vi "HVACmotes.vi"() -> ()   [LabVIEW 2011]
uses:
  <vilib>/picture/picture.llb/Draw True-Color Pixmap.vi
panel:
  out "CO2":dbl(graph)
  out "Node ID":u8
  out "Light":dbl(graph)
  out "Humidity":dbl(graph)
  out "Temperature":dbl(graph)
  in  "header size":i32=9
  in  "bytes to read":i32=10
  out "Packet Payload":string
  in  "Enable Read":bool=TRUE
  in  "Port Number":i32=9002
  out "KTH  Automatic Control \nTemplates. Read from SerialForwarder":picture
  # "For TestSerialCommMsg:\nheaderSize = 9\npayload = 10"
  # "Communication control"
  # "Communication results"
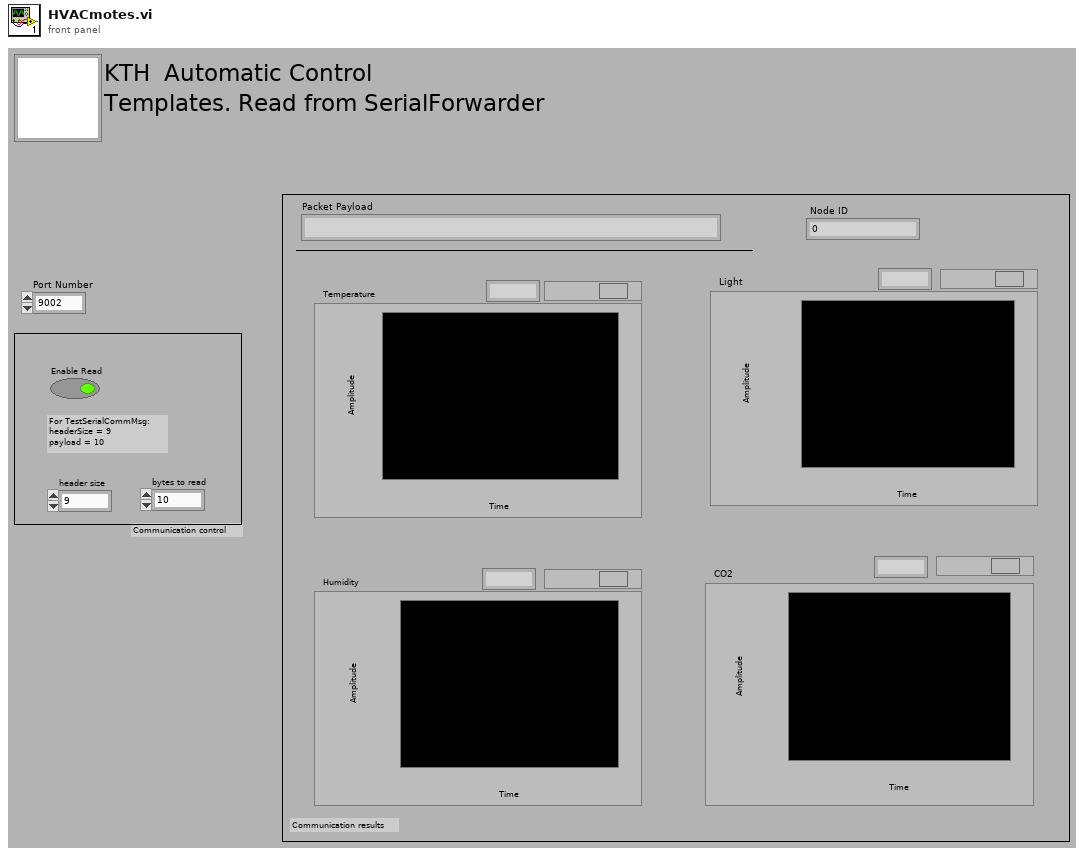
[diagram p1: front panel]
types:
  T1 = typedef "imagedata.ctl" = cluster{"image type":i32, "image depth":i32, "image":u8[], "mask":u8[], "colors":u32[], "Rectangle":cluster{"left":i16, "top":i16, "right":i16, "bottom":i16}}
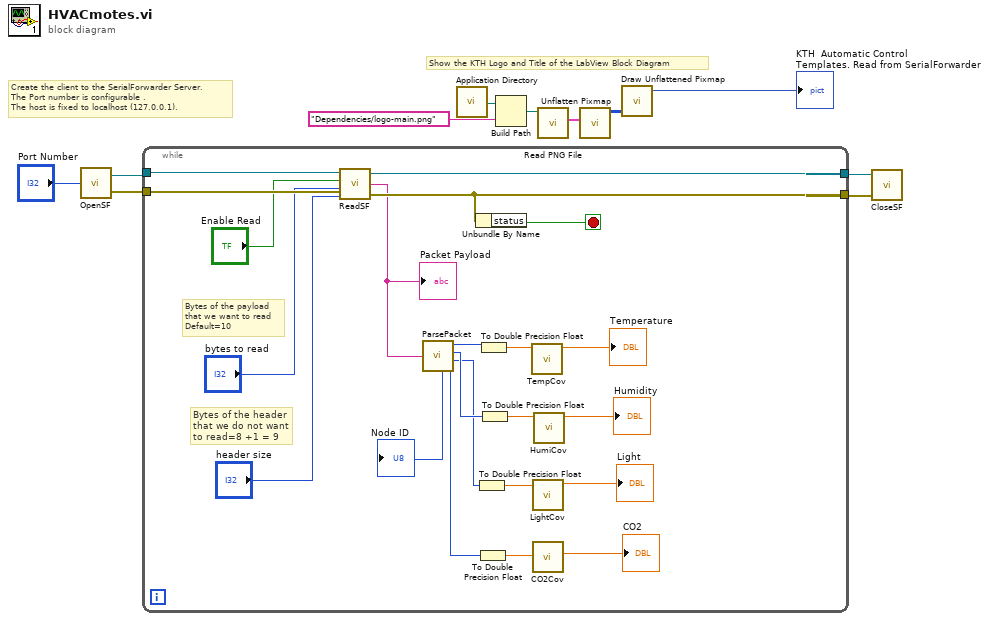
[diagram p0: block diagram]
diagram:
  # "Create the client to the SerialForwarder Server.\nThe Port number is configurable . \nThe host is fixed to localhost (127.0.0.1)."
  # "Show the KTH Logo and Title of the LabView Block Diagram"
  n1 = call "OpenSF.vi"("Port Number"="Port Number") -> ("error out"=w10:errorcluster, "connection ID"=w11:refnum<k5>)
  n2 = while {
    tunnel: w11 -> [w32]
    tunnel: w10 -> [w33]
    tunnel: [w31] -> w9
    tunnel: [w29] -> w8
    stop <- w30 stop-if-true
    # "Bytes of the payload \nthat we want to read\nDefault=10"
    # "Bytes of the header\nthat we do not want \nto read=8 +1 = 9"
    n3 = call "ReadSF.vi"("connection ID in"=w32, "error in"=w33, "enabled"="Enable Read", "bytes to read"="bytes to read", "header size"="header size") -> ("connection ID out"=w31:refnum<k5>, "string"=w25:string, "error out"=w29:errorcluster)  [unwired: 1 in]
    "Packet Payload" <- w25
    n4 = call "ParsePacket.vi"("data out"=w25) -> ("Node ID"=→"Node ID":u8, "CO2"=w15:u16, "Light"=w16:u16, "Humidity"=w17:u16, "Temperature"=w24:u16)  [unwired: 1 out]
    n5 = Unbundle By Name(w29) -> ("status"=w30:bool)
    n6 = To Double Precision Float(number=w16) -> (double precision float=w19:dbl)
    n7 = To Double Precision Float(number=w15) -> (double precision float=w14:dbl)
    n8 = To Double Precision Float(number=w24) -> (double precision float=w23:dbl)
    n9 = To Double Precision Float(number=w17) -> (double precision float=w21:dbl)
    n10 = call "TempCov.vi"("Input x"=w23) -> ("Temperature"=→"Temperature":dbl)  [unwired: 10 in]
    n11 = call "LightCov.vi"("Input x"=w19) -> ("Light"=→"Light":dbl)  [unwired: 10 in]
    n12 = call "CO2Cov.vi"("Input x"=w14) -> ("CO2"=→"CO2":dbl)  [unwired: 9 in]
    n13 = call "HumiCov.vi"("Input x"=w21) -> ("Humidity"=→"Humidity":dbl)  [unwired: 10 in]
  }
  n14 = call <vilib>:"Application Directory.vi"() -> ("Application Directory"=w3:path)
  n15 = Build Path(base path=w3, name or relative path="Dependencies/logo-main.png") -> (appended path=w4:path)
  n16 = call <vilib>:"Read PNG File.vi"("path to PNG file"=w4) -> ("image data"=w7:T1)  [unwired: 8 in, 2 out]
  n17 = call <vilib>:"Unflatten Pixmap.vi"("image data"=w7) -> ("24-bit pixmap"=w6:u32[][])  [unwired: 4 in, 6 out]
  n18 = call-poly <vilib>:"Draw Unflattened Pixmap.vi"("data (RGB format)"=w6) -> ("new picture"=→"KTH  Automatic Control \nTemplates. Read from SerialForwarder":picture)  [unwired: 8 in]
  n19 = call "CloseSF.vi"("error out"=w8, "connection ID"=w9) -> ()  [unwired: 1 in]
